vi "HoloPy_get_sum_bin_planes.vi"(8 "error in (no error)":errorcluster, 11 "Refnum in":refnum<k35>) -> (0 "error out":errorcluster, 2 "XY Plane":i32[][](array[numeric]), 3 "Refnum out":refnum<k35>)   [LabVIEW 2025, in "holoTracker.lvlib"]
uses:
  holoTracker.lvlib
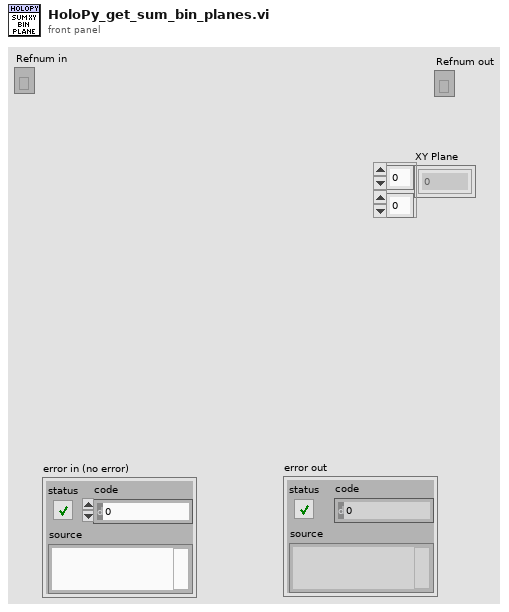
[diagram p1: front panel]
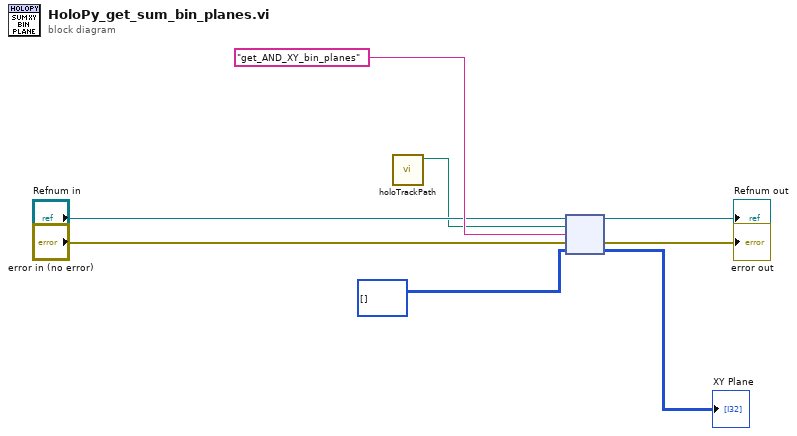
[diagram p0: block diagram]
diagram:
  n1 = call "holoTrackPath.vi"() -> ("appended path"=w1:path)  [unwired: 11 in]
  n2 = node("Refnum in", w1, "get_AND_XY_bin_planes" ("function name"), "error in (no error)", i32[][] []) -> (→"Refnum out":refnum<k35>, →"error out":errorcluster, →"XY Plane":i32[][])  [unwired: 2 out]
